vi "subFindProjects.vi"(11 "SolutionBuilder in":refnum<class "SolutionBuilder.lvclass">) -> (3 "SolutionBuilder out":refnum<class "SolutionBuilder.lvclass">)   [LabVIEW 2020, in "SolutionBuilder.lvlib" / "SolutionBuilder.lvclass"]
uses:
  SolutionBuilder.lvclass
  <vilib>/xml/Load XML File.vi
  <vilib>/xml/Close Reference(Node).vi
  <vilib>/regexp/Match Regular Expression.xnode
  <vilib>/xml/NI_XML.lvlib
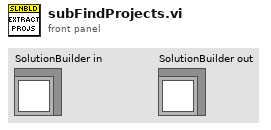
[diagram p1: front panel]
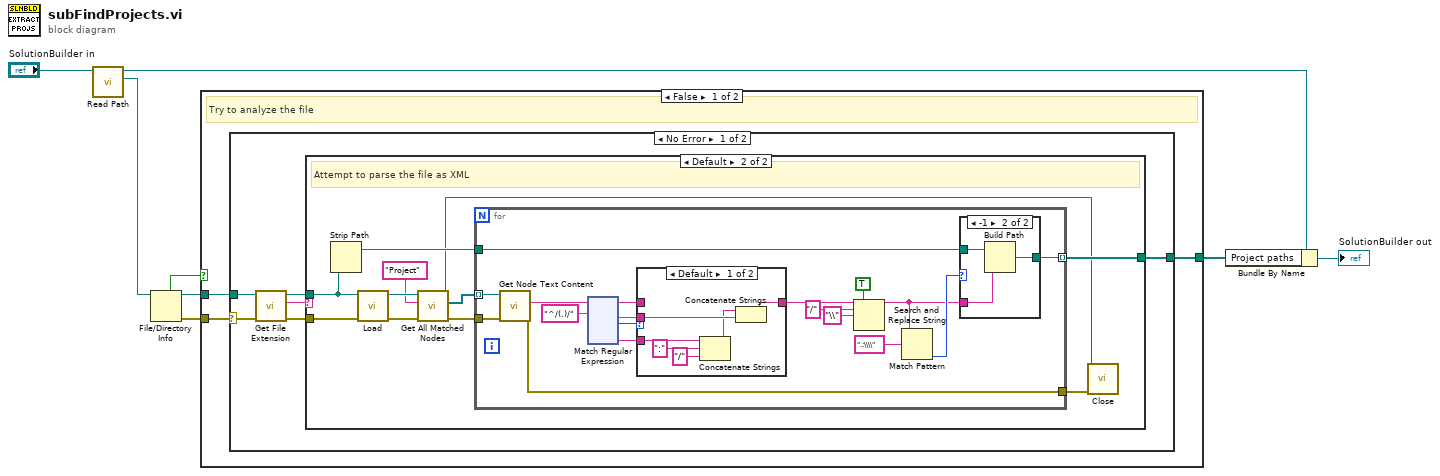
[diagram p0: block diagram]
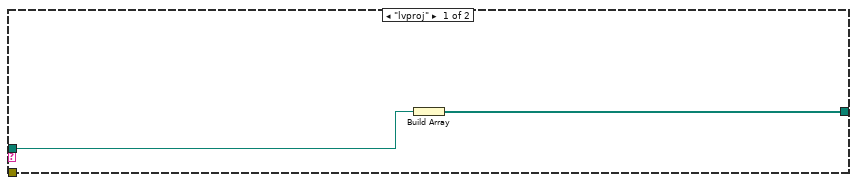
[diagram p2: hidden frame]
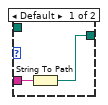
[diagram p4: hidden frame]
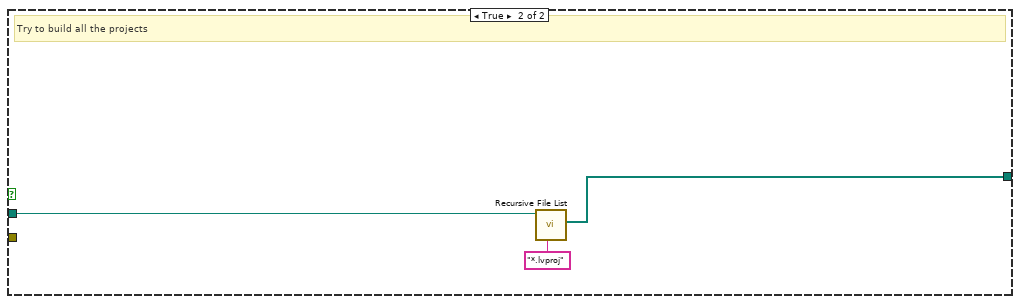
[diagram p6: hidden frame]
diagram:
  n1 = call-dynamic "Read Path.vi"("SolutionBuilder in"="SolutionBuilder in") -> ("Path"=w4:path, "SolutionBuilder out"=w3:refnum<class "SolutionBuilder.lvclass">)  [unwired: 9 in]
  n2 = File/Directory Info(path=w4) -> (path out=w7:path, directory=w8:bool, error out=w6:errorcluster)  [unwired: 1 in, 4 out]
  n3 = case shown="False" w8 {
    tunnel: [w9 w178] -> w2
    tunnel: w7 -> [w11 w177]
    tunnel: w6 -> [w10 _]
    frame False {
      # "Try to analyze the file"
      n4 = case shown="No Error" w10 {
        selector: w10 -> [w16 _]
        tunnel: w11 -> [w15 _]
        tunnel: [w17 _] -> w9
        frame No Error {
          n5 = call <vilib>:"Get File Extension.vi"("error in (no error)"=w16, "file"=w15) -> ("error out"=w13:errorcluster, "lowercase file extension"=w12:string, "dup file"=w14:path)  [unwired: 5 in, 2 out]
          n6 = case shown="Default" w12 {
            tunnel: [w18 w24] -> w17
            tunnel: w14 -> [w19 w21]
            tunnel: w13 -> [_ w20]
            frame "lvproj" {
              n7 = Build Array(w19) -> (w18:path[])
            }
            frame Default {
              # "Attempt to parse the file as XML"
              n8 = Strip Path(path=w21) -> (stripped path=w25:path)  [unwired: 1 out]
              n9 = call-poly <vilib>:"Load.vi"("path to XML document"=w21, "error in (no error)"=w20) -> ("DOM document out"=w30:refnum<k20>, "error out"=w29:errorcluster)  [unwired: 11 in, 1 out]
              n10 = call <vilib>:"Get All Matched Nodes.vi"("error in (no error)"=w29, "XPath expression"="Project", "node in"=w30) -> ("error out"=w27:errorcluster, "node result array"=w26:refnum<k20>[], "node out"=w22:refnum<k20>)  [unwired: 6 in]
              n11 = for {
                tunnel: w27 -> [w48]
                tunnel: w26 -> [w47] mode=indexing
                tunnel: [w43] -> w24 mode=indexing
                tunnel: w25 -> [w44]
                tunnel: [w31] -> w23
                n12 = call <vilib>:"Get Node Text Content.vi"("error in (no error)"=w48, "node in"=w47) -> ("error out"=w31:errorcluster, "node text"=w42:string)  [unwired: 7 in, 1 out]
                n13 = xnode "Match Regular Expression"("input string"=w42, "regular expression"="^/(.)/") -> ("before match"=w39:string, "after match"=w37:string, "offset past match"=w40:i32, "submatch 1"=w38:string)  [unwired: 4 in, 2 out]
                n14 = case shown="Default" w40 {
                  tunnel: w39 -> [_ w55]
                  tunnel: [w51 w55] -> w36
                  tunnel: w38 -> [w53 _]
                  tunnel: w37 -> [w54 _]
                  frame Default {
                    n15 = Concatenate Strings(w53, ":" ("string"), "/" ("string")) -> (w50:string)
                    n16 = Concatenate Strings(w50, w54) -> (w51:string)
                  }
                  frame -1 {
                  }
                }
                n17 = Search and Replace String(replace all?=TRUE ("replace all? (F)"), input string=w36, search string="/", replace string="\\" ("replace string (\"\")")) -> (result string=w35:string)  [unwired: 4 in, 3 out]
                n18 = Match Pattern(string=w35, regular expression=".:\\\\") -> (offset past match=w45:i32)  [unwired: 1 in, 3 out]
                n19 = case shown="-1" w45 {
                  tunnel: w44 -> [_ w176]
                  tunnel: w35 -> [w172 w175]
                  tunnel: [w173 w174] -> w43
                  frame Default {
                    n20 = String To Path(string=w172) -> (path=w173:path)
                  }
                  frame -1 {
                    n21 = Build Path(base path=w176, name or relative path=w175) -> (appended path=w174:path)
                  }
                }
              }
              n22 = call-poly <vilib>:"Close.vi"("error in (no error)"=w23, "node"=w22) -> ()  [unwired: 7 in, 1 out]
            }
          }
        }
        frame Error {
        }
      }
    }
    frame True {
      # "Try to build all the projects"
      n23 = call <vilib>:"Recursive File List.vi"("pattern"="*.lvproj", "Folder Path"=w177) -> ("All Files in Dir"=w178:path[])  [unwired: 5 in, 4 out]
    }
  }
  n24 = Bundle By Name(cluster=w3, "Project paths"=w2) -> (→"SolutionBuilder out":refnum<class "SolutionBuilder.lvclass">)
